vi "Config OK Tab.vi"(8 "error in (no error)":errorcluster, 9 "String Selected":T1, 11 "Rigol DG822 Square in":refnum<class "Rigol DG822 Square.lvclass">) -> (0 "error out":errorcluster, 3 "Rigol DG822 Square out":refnum<class "Rigol DG822 Square.lvclass">)   [LabVIEW 2021, in "Rigol DG822 UI.lvlib" / "Rigol DG822 Square.lvlib" / "Rigol DG822 Square.lvclass"]
uses:
  Rigol DG822 Square.lvclass
  Rigol DG822 UI/lib/controls.llb/StringIndicatorSelected.ctl
  Rigol DG822 Square.lvclass/Rigol DG822 Square.ctl
  General/Files/lvlibp/Actors.lvlibp/Actors/Actors/Actors.lvclass
  D:/LabVIEW/General/Files/lvlibp/Actors.lvlibp/Actors/Actors/Actors.lvclass
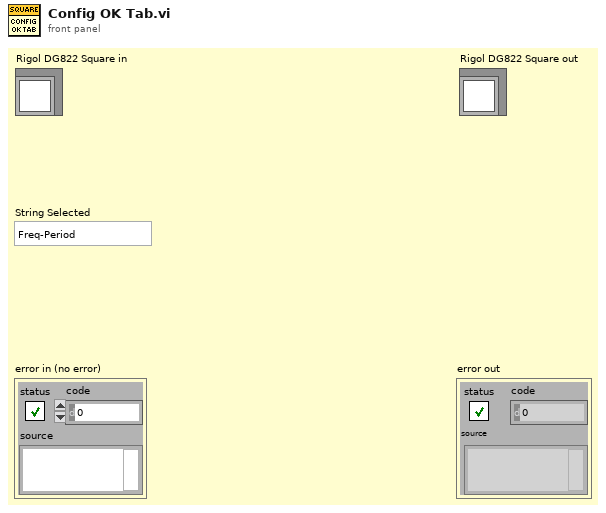
[diagram p1: front panel]
types:
  T1 = typedef "StringIndicatorSelected.ctl" = enum16{"Freq-Period", "Ampl-HighL", "Offset-LowL", "Phase", "Duty-Width", "RisEdge", "FallEdge"}
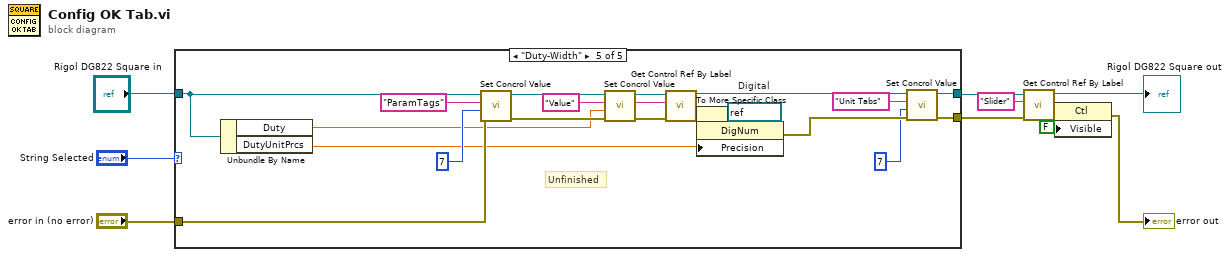
[diagram p0: block diagram]
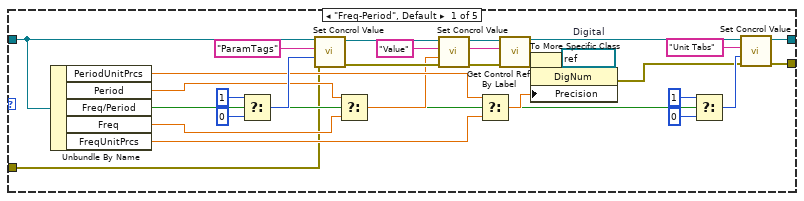
[diagram p2: hidden frame]
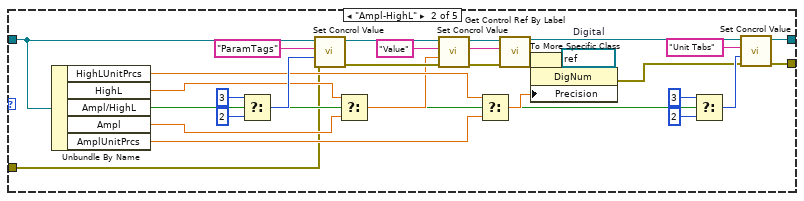
[diagram p3: hidden frame]
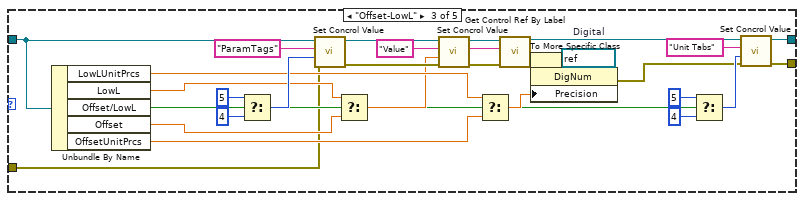
[diagram p4: hidden frame]
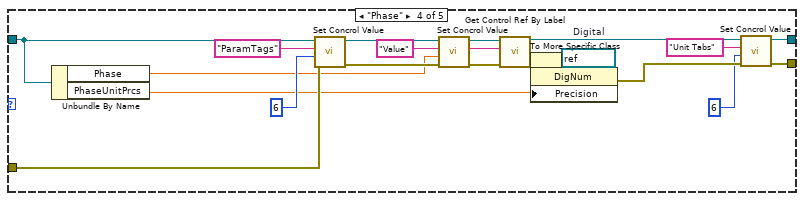
[diagram p5: hidden frame]
diagram:
  n1 = case shown="\"Duty-Width\"" "String Selected" {
    tunnel: [w17 w47 w78 w112 w134] -> w3
    tunnel: "Rigol DG822 Square in" -> [w13 w60 w91 w119 w141]
    tunnel: [w14 w43 w74 w109 w131] -> w1
    tunnel: "error in (no error)" -> [w15 w44 w75 w110 w132]
    frame "Freq-Period", Default {
      w35 = refnum<vi> refnum  # Digital
      w26 = "Value" ("Control Label")
      n2 = Unbundle By Name(w13) -> ("PeriodUnitPrcs"=w20:dbl, "Period"=w23:dbl, "Freq/Period"=w16:bool, "Freq"=w22:dbl, "FreqUnitPrcs"=w21:dbl)
      n3 = Select(t=u16 1 ("ParamTags"), s=w16, f=u16 0 ("ParamTags")) -> (s? t:f=w27:u16)
      n4 = call "Set Concrol Value.vi"("error in (no error)"=w15, "Value"=w27, "Control Label"="ParamTags", "Actors in"=w13) -> ("error out"=w25:errorcluster, "Actors out"=w29:refnum<class "Rigol DG822 Square.lvclass">)  [unwired: 6 in]
      n5 = Select(t=w23, s=w16, f=w22) -> (s? t:f=w19:dbl)
      n6 = call "Set Concrol Value.vi"("error in (no error)"=w25, "Value"=w19, "Control Label"=w26, "Actors in"=w29) -> ("error out"=w24:errorcluster, "Actors out"=w28:refnum<class "Rigol DG822 Square.lvclass">)  [unwired: 6 in]
      n7 = Select(t=w20, s=w16, f=w21) -> (s? t:f=w36:dbl)
      n8 = call "Get Control Ref By Label.vi"("error in (no error)"=w24, "Control Label"=w26, "Actors in"=w28) -> ("error out"=w37:errorcluster, "Control Ref"=w33:refnum<vi>, "Actors out"=w18:refnum<class "Rigol DG822 Square.lvclass">)  [unwired: 6 in]
      n9 = To More Specific Class(target class=w35, reference=w33, error in=w37) -> (specific class reference=w34:refnum<vi>, error out=w38:errorcluster)
      n10 = property class="DigNum"(reference=w34, error in=w38, "Precision"=w36) -> (error out=w12:errorcluster)  [unwired: 1 out]
      n11 = Select(t=u16 1 ("ParamTags"), s=w16, f=u16 0 ("ParamTags")) -> (s? t:f=w42:u16)
      n12 = call "Set Concrol Value.vi"("error in (no error)"=w12, "Value"=w42, "Control Label"="Unit Tabs", "Actors in"=w18) -> ("error out"=w14:errorcluster, "Actors out"=w17:refnum<class "Rigol DG822 Square.lvclass">)  [unwired: 6 in]
    }
    frame "Ampl-HighL" {
      w66 = refnum<vi> refnum  # Digital
      w56 = "Value" ("Control Label")
      n13 = Unbundle By Name(w60) -> ("HighLUnitPrcs"=w50:dbl, "HighL"=w53:dbl, "Ampl/HighL"=w45:bool, "Ampl"=w52:dbl, "AmplUnitPrcs"=w51:dbl)
      n14 = Select(t=u16 3 ("ParamTags"), s=w45, f=u16 2 ("ParamTags")) -> (s? t:f=w57:u16)
      n15 = call "Set Concrol Value.vi"("error in (no error)"=w44, "Value"=w57, "Control Label"="ParamTags", "Actors in"=w60) -> ("error out"=w55:errorcluster, "Actors out"=w59:refnum<class "Rigol DG822 Square.lvclass">)  [unwired: 6 in]
      n16 = Select(t=w53, s=w45, f=w52) -> (s? t:f=w49:dbl)
      n17 = call "Set Concrol Value.vi"("error in (no error)"=w55, "Value"=w49, "Control Label"=w56, "Actors in"=w59) -> ("error out"=w54:errorcluster, "Actors out"=w58:refnum<class "Rigol DG822 Square.lvclass">)  [unwired: 6 in]
      n18 = Select(t=w50, s=w45, f=w51) -> (s? t:f=w67:dbl)
      n19 = call "Get Control Ref By Label.vi"("error in (no error)"=w54, "Control Label"=w56, "Actors in"=w58) -> ("error out"=w68:errorcluster, "Control Ref"=w64:refnum<vi>, "Actors out"=w48:refnum<class "Rigol DG822 Square.lvclass">)  [unwired: 6 in]
      n20 = To More Specific Class(target class=w66, reference=w64, error in=w68) -> (specific class reference=w65:refnum<vi>, error out=w69:errorcluster)
      n21 = property class="DigNum"(reference=w65, error in=w69, "Precision"=w67) -> (error out=w46:errorcluster)  [unwired: 1 out]
      n22 = Select(t=u16 3 ("ParamTags"), s=w45, f=u16 2 ("ParamTags")) -> (s? t:f=w73:u16)
      n23 = call "Set Concrol Value.vi"("error in (no error)"=w46, "Value"=w73, "Control Label"="Unit Tabs", "Actors in"=w48) -> ("error out"=w43:errorcluster, "Actors out"=w47:refnum<class "Rigol DG822 Square.lvclass">)  [unwired: 6 in]
    }
    frame "Offset-LowL" {
      w97 = refnum<vi> refnum  # Digital
      w87 = "Value" ("Control Label")
      n24 = Unbundle By Name(w91) -> ("LowLUnitPrcs"=w81:dbl, "LowL"=w84:dbl, "Offset/LowL"=w76:bool, "Offset"=w83:dbl, "OffsetUnitPrcs"=w82:dbl)
      n25 = Select(t=u16 5 ("ParamTags"), s=w76, f=u16 4 ("ParamTags")) -> (s? t:f=w88:u16)
      n26 = call "Set Concrol Value.vi"("error in (no error)"=w75, "Value"=w88, "Control Label"="ParamTags", "Actors in"=w91) -> ("error out"=w86:errorcluster, "Actors out"=w90:refnum<class "Rigol DG822 Square.lvclass">)  [unwired: 6 in]
      n27 = Select(t=w84, s=w76, f=w83) -> (s? t:f=w80:dbl)
      n28 = call "Set Concrol Value.vi"("error in (no error)"=w86, "Value"=w80, "Control Label"=w87, "Actors in"=w90) -> ("error out"=w85:errorcluster, "Actors out"=w89:refnum<class "Rigol DG822 Square.lvclass">)  [unwired: 6 in]
      n29 = Select(t=w81, s=w76, f=w82) -> (s? t:f=w98:dbl)
      n30 = call "Get Control Ref By Label.vi"("error in (no error)"=w85, "Control Label"=w87, "Actors in"=w89) -> ("error out"=w99:errorcluster, "Control Ref"=w95:refnum<vi>, "Actors out"=w79:refnum<class "Rigol DG822 Square.lvclass">)  [unwired: 6 in]
      n31 = To More Specific Class(target class=w97, reference=w95, error in=w99) -> (specific class reference=w96:refnum<vi>, error out=w100:errorcluster)
      n32 = property class="DigNum"(reference=w96, error in=w100, "Precision"=w98) -> (error out=w77:errorcluster)  [unwired: 1 out]
      n33 = Select(t=u16 5 ("ParamTags"), s=w76, f=u16 4 ("ParamTags")) -> (s? t:f=w104:u16)
      n34 = call "Set Concrol Value.vi"("error in (no error)"=w77, "Value"=w104, "Control Label"="Unit Tabs", "Actors in"=w79) -> ("error out"=w74:errorcluster, "Actors out"=w78:refnum<class "Rigol DG822 Square.lvclass">)  [unwired: 6 in]
    }
    frame "Phase" {
      w123 = refnum<vi> refnum  # Digital
      w116 = "Value" ("Control Label")
      n35 = Unbundle By Name(w119) -> ("Phase"=w107:dbl, "PhaseUnitPrcs"=w106:dbl)
      n36 = call "Set Concrol Value.vi"("error in (no error)"=w110, "Value"=u16 6 ("ParamTags"), "Control Label"="ParamTags", "Actors in"=w119) -> ("error out"=w115:errorcluster, "Actors out"=w118:refnum<class "Rigol DG822 Square.lvclass">)  [unwired: 6 in]
      n37 = call "Set Concrol Value.vi"("error in (no error)"=w115, "Value"=w107, "Control Label"=w116, "Actors in"=w118) -> ("error out"=w114:errorcluster, "Actors out"=w117:refnum<class "Rigol DG822 Square.lvclass">)  [unwired: 6 in]
      n38 = call "Get Control Ref By Label.vi"("error in (no error)"=w114, "Control Label"=w116, "Actors in"=w117) -> ("error out"=w124:errorcluster, "Control Ref"=w121:refnum<vi>, "Actors out"=w113:refnum<class "Rigol DG822 Square.lvclass">)  [unwired: 6 in]
      n39 = To More Specific Class(target class=w123, reference=w121, error in=w124) -> (specific class reference=w122:refnum<vi>, error out=w125:errorcluster)
      n40 = property class="DigNum"(reference=w122, error in=w125, "Precision"=w106) -> (error out=w111:errorcluster)  [unwired: 1 out]
      n41 = call "Set Concrol Value.vi"("error in (no error)"=w111, "Value"=u16 6 ("ParamTags"), "Control Label"="Unit Tabs", "Actors in"=w113) -> ("error out"=w109:errorcluster, "Actors out"=w112:refnum<class "Rigol DG822 Square.lvclass">)  [unwired: 6 in]
    }
    frame "Duty-Width" {
      w145 = refnum<vi> refnum  # Digital
      w138 = "Value" ("Control Label")
      # "Unfinished"
      n42 = Unbundle By Name(w141) -> ("Duty"=w129:dbl, "DutyUnitPrcs"=w128:dbl)
      n43 = call "Set Concrol Value.vi"("error in (no error)"=w132, "Value"=u16 7 ("ParamTags"), "Control Label"="ParamTags", "Actors in"=w141) -> ("error out"=w137:errorcluster, "Actors out"=w140:refnum<class "Rigol DG822 Square.lvclass">)  [unwired: 6 in]
      n44 = call "Set Concrol Value.vi"("error in (no error)"=w137, "Value"=w129, "Control Label"=w138, "Actors in"=w140) -> ("error out"=w136:errorcluster, "Actors out"=w139:refnum<class "Rigol DG822 Square.lvclass">)  [unwired: 6 in]
      n45 = call "Get Control Ref By Label.vi"("error in (no error)"=w136, "Control Label"=w138, "Actors in"=w139) -> ("error out"=w146:errorcluster, "Control Ref"=w143:refnum<vi>, "Actors out"=w135:refnum<class "Rigol DG822 Square.lvclass">)  [unwired: 6 in]
      n46 = To More Specific Class(target class=w145, reference=w143, error in=w146) -> (specific class reference=w144:refnum<vi>, error out=w147:errorcluster)
      n47 = property class="DigNum"(reference=w144, error in=w147, "Precision"=w128) -> (error out=w133:errorcluster)  [unwired: 1 out]
      n48 = call "Set Concrol Value.vi"("error in (no error)"=w133, "Value"=u16 7 ("ParamTags"), "Control Label"="Unit Tabs", "Actors in"=w135) -> ("error out"=w131:errorcluster, "Actors out"=w134:refnum<class "Rigol DG822 Square.lvclass">)  [unwired: 6 in]
    }
  }
  n49 = call "Get Control Ref By Label.vi"("error in (no error)"=w1, "Control Label"="Slider", "Actors in"=w3) -> ("error out"=w6:errorcluster, "Control Ref"=w5:refnum<vi>, "Actors out"=→"Rigol DG822 Square out":refnum<class "Rigol DG822 Square.lvclass">)  [unwired: 6 in]
  n50 = property class="Ctl"(reference=w5, error in=w6, "Visible"=FALSE) -> (error out=→"error out":errorcluster)  [unwired: 1 out]
